vi "Index 3D Array (returns 1D Array)_.vi"(8 "1D array \n(index < 0)":dbl[](array[numeric]), 9 "index":i32=-1, 10 "3D array":dbl[][][](array[numeric])=[[[0.0], [0.0], [0.0]], [[1.0], [1.0], [1.0]]]) -> (2 "1D array":dbl[](array[numeric]))   [LabVIEW 2014]
doc: "Use this template to build a VI to use as a subVI."
panel:
  in  "?":enum32{"3D Array", "1D Array"}(tab)
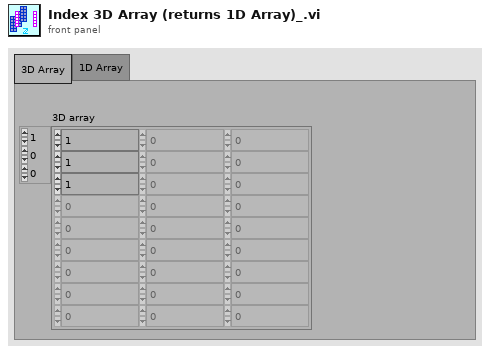
[diagram p1: front panel]
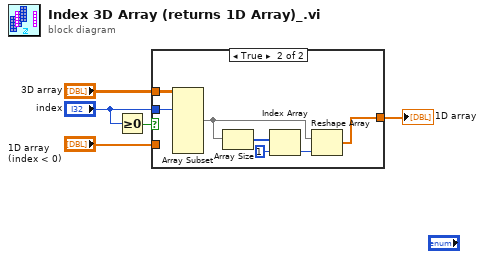
[diagram p0: block diagram]
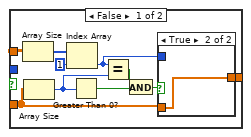
[diagram p2: hidden frame]
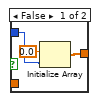
[diagram p3: hidden frame]
diagram:
  n1 = Greater Or Equal To 0?(x="index") -> (x >= 0?=w3:bool)
  n2 = case shown="True" w3 {
    tunnel: [w6 w26] -> w5
    tunnel: "3D array" -> [w12 w25]
    tunnel: "index" -> [_ w24]
    tunnel: "1D array \n(index < 0)" -> [w15 _]
    frame False {
      n3 = Array Size(array=w12) -> (size(s)=w13:i32[])
      n4 = Array Size(array=w15) -> (size(s)=w8:i32)
      n5 = Index Array(array=w13, index=1) -> (element=w9:i32)
      n6 = Greater Than 0?(x=w8) -> (x > 0?=w10:bool)
      n7 = Equal?(x=w9, y=w8) -> (x = y?=w7:bool)
      n8 = And(x=w7, y=w10) -> (x .and. y?=w11:bool)
      n9 = case shown="True" w11 {
        tunnel: w15 -> [_ w19]
        tunnel: w9 -> [w17 _]
        tunnel: [w16 w19] -> w6
        frame False {
          n10 = Initialize Array(0.0 ("element"), w17) -> (w16:dbl[])
        }
        frame True {
        }
      }
    }
    frame True {
      n11 = Array Subset(array=w25, index (dim 0)=w24) -> (w20:dbl[][][])  [unwired: 5 in]
      n12 = Array Size(array=w20) -> (size(s)=w21:i32[])
      n13 = Index Array(array=w21, index=1) -> (element=w23:i32)
      n14 = Reshape Array(w20, w23) -> (w26:dbl[])
    }
  }
  "1D array" <- w5
